vi "pl1000Stop.vi"(8 "error in (no error)":errorcluster, 11 "pl1000 handle":i16) -> (0 "error out":errorcluster, 3 "pl1000 handle out":i16)   [LabVIEW 2016, in "pl1000.lvlib"]
doc: "This function aborts data collection."
uses:
  pl1000.lvlib
  pl1000.dll
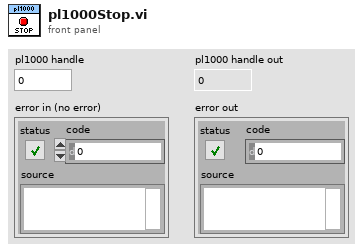
[diagram p1: front panel]
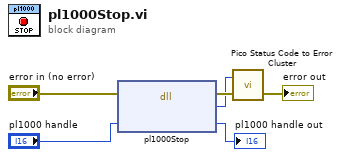
[diagram p0: block diagram]
diagram:
  n1 = dll-call lib="pl1000.dll" fn="pl1000Stop"(error in="error in (no error)", "handle"="pl1000 handle") -> (error out=w4:errorcluster, "status"=w3:u32, "handle"=→"pl1000 handle out":i16)  [unwired: 2 in, 1 out]
  n2 = call "Pico Status Code to Error Cluster.vi"("error in"=w4, "PICO_STATUS"=w3) -> ("error out"=→"error out":errorcluster)  [unwired: 1 in]
